vi "programa6.vi"() -> ()   [LabVIEW 2011]
uses:
  le/Control 2.ctl
  <vilib>/express/express arith-compare/Formula/XNode/ExpressFormulaBlockNode.xnode
panel:
  out "Array 2":string[](array[string])
  out "Array":dbl[](array[numeric])
  # "En el arreglo 1 ingresar 5 numeros enteros y luego en el arreglo 2\n escribir si es par o impar cada uno de los numeros."
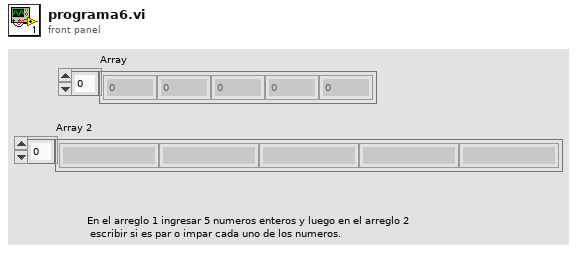
[diagram p1: front panel]
types:
  T1 = typedef "Control 2.ctl" = enum16{"iniciar arreglos", "rellenar arreglo1", "encontrarPareImpares", "final"}
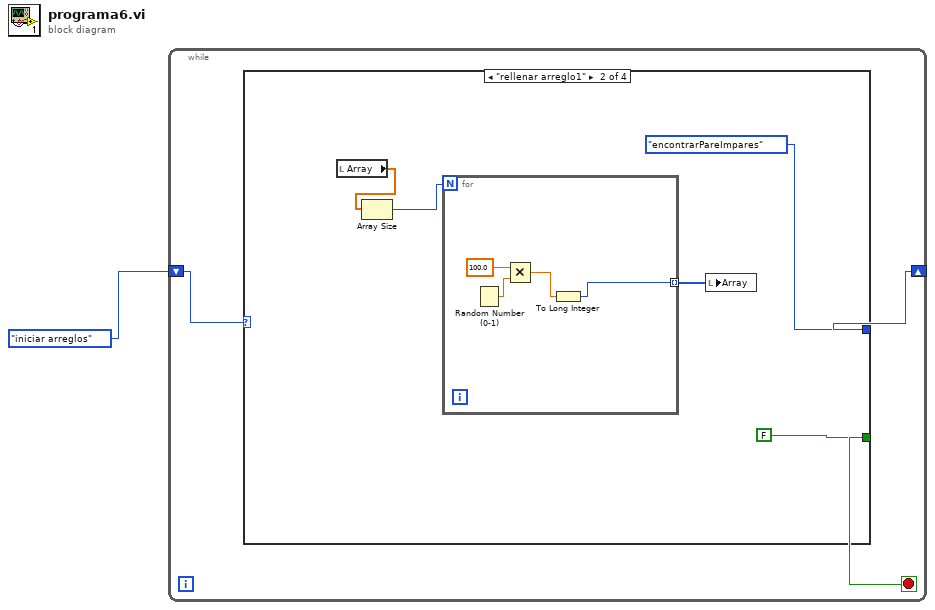
[diagram p0: block diagram]
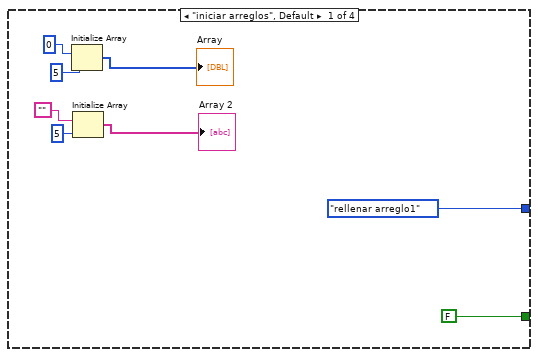
[diagram p2: hidden frame]
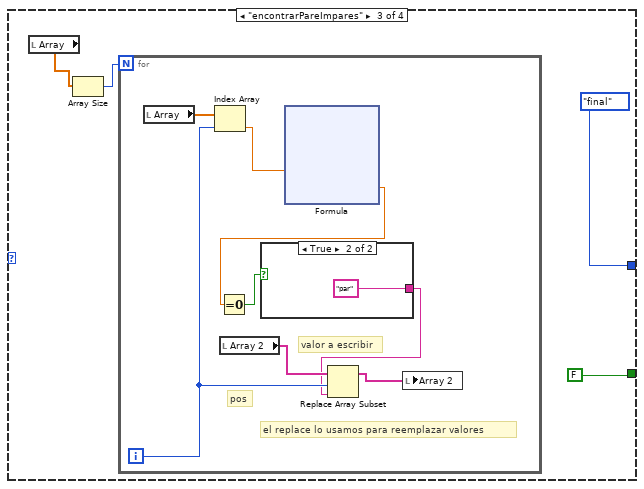
[diagram p3: hidden frame]
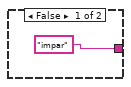
[diagram p4: hidden frame]
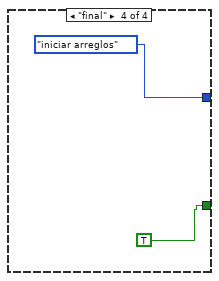
[diagram p5: hidden frame]
diagram:
  n1 = while {
    shift-right: [w3] -> _
    shift-left: Control_2."iniciar arreglos" -> [w4]
    stop <- w2 stop-if-true
    n2 = case shown="\"rellenar arreglo1\"" w4 {
      tunnel: [Control_2."rellenar arreglo1" Control_2."encontrarPareImpares" Control_2."final" Control_2."iniciar arreglos"] -> w3
      tunnel: [FALSE FALSE FALSE TRUE] -> w2
      frame "iniciar arreglos", Default {
        n3 = Initialize Array(0, 5 ("dimension size")) -> (→"Array":i32[])
        n4 = Initialize Array("", 5 ("dimension size")) -> (→"Array 2":string[])
      }
      frame "rellenar arreglo1" {
        n5 = local read "Array"() -> (w17:dbl[])
        n6 = Array Size(array=w17) -> (size(s)=w16:i32)
        n7 = for {
          N: w16 -> [_]
          tunnel: [w18] -> w15 mode=indexing
          n8 = Random Number (0-1)() -> (number: 0 to 1=w20:dbl)
          n9 = Multiply(x=100.0, y=w20) -> (x*y=w19:dbl)
          n10 = To Long Integer(number=w19) -> (32bit integer=w18:i32)
        }
        n11 = local write "Array"(w15) -> ()
      }
      frame "encontrarPareImpares" {
        n12 = local read "Array"() -> (w25:dbl[])
        n13 = Array Size(array=w25) -> (size(s)=w24:i32)
        n14 = for {
          N: w24 -> [_]
          i -> [w28]
          # "pos"
          # "el replace lo usamos para reemplazar valores"
          # "valor a escribir"
          n15 = local read "Array"() -> (w33:dbl[])
          n16 = Index Array(array=w33, index=w28) -> (element=w32:dbl)
          n17 = local read "Array 2"() -> (w29:string[])
          n18 = xnode "Formula"("X1"=w32) -> ("Result"=w30:dbl)  [unwired: 1 in, 1 out]
          n19 = Equal To 0?(x=w30) -> (x = 0?=w31:bool)
          n20 = case shown="True" w31 {
            tunnel: ["impar" "par"] -> w26
            frame False {
            }
            frame True {
            }
          }
          n21 = Replace Array Subset(array=w29, new element=w26, index=w28) -> (w27:string[])
          n22 = local write "Array 2"(w27) -> ()
        }
      }
      frame "final" {
      }
    }
  }
